vi "DAQ - 1-7 Modules - SubVI.vi"(11 "array":dbl[](array[numeric])) -> (3 "output array":dbl[](array[numeric]))   [LabVIEW 2015]
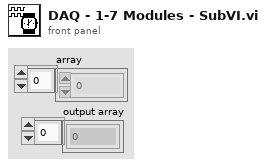
[diagram p1: front panel]
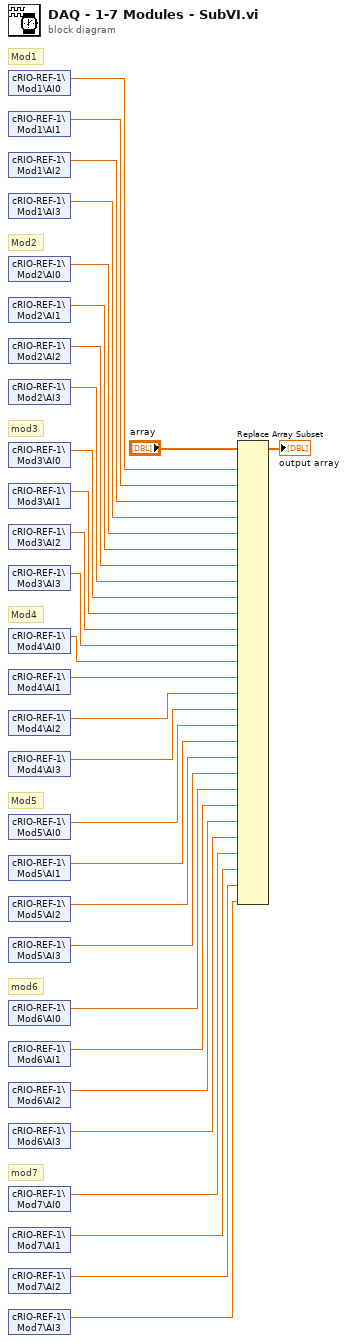
[diagram p0: block diagram]
diagram:
  # "mod3"
  # "Mod1"
  # "Mod2"
  # "mod6"
  # "mod7"
  # "Mod4"
  # "Mod5"
  n1 = shared-variable "cRIO-REF-1\\Mod1\\AI0"() -> (w1:dbl)  [unwired: 1 in, 1 out]
  n2 = shared-variable "cRIO-REF-1\\Mod1\\AI1"() -> (w2:dbl)  [unwired: 1 in, 1 out]
  n3 = shared-variable "cRIO-REF-1\\Mod1\\AI2"() -> (w3:dbl)  [unwired: 1 in, 1 out]
  n4 = shared-variable "cRIO-REF-1\\Mod1\\AI3"() -> (w4:dbl)  [unwired: 1 in, 1 out]
  n5 = shared-variable "cRIO-REF-1\\Mod2\\AI0"() -> (w5:dbl)  [unwired: 1 in, 1 out]
  n6 = shared-variable "cRIO-REF-1\\Mod2\\AI1"() -> (w6:dbl)  [unwired: 1 in, 1 out]
  n7 = shared-variable "cRIO-REF-1\\Mod2\\AI2"() -> (w7:dbl)  [unwired: 1 in, 1 out]
  n8 = shared-variable "cRIO-REF-1\\Mod2\\AI3"() -> (w8:dbl)  [unwired: 1 in, 1 out]
  n9 = shared-variable "cRIO-REF-1\\Mod3\\AI0"() -> (w9:dbl)  [unwired: 1 in, 1 out]
  n10 = shared-variable "cRIO-REF-1\\Mod3\\AI1"() -> (w10:dbl)  [unwired: 1 in, 1 out]
  n11 = shared-variable "cRIO-REF-1\\Mod3\\AI2"() -> (w11:dbl)  [unwired: 1 in, 1 out]
  n12 = shared-variable "cRIO-REF-1\\Mod3\\AI3"() -> (w12:dbl)  [unwired: 1 in, 1 out]
  n13 = shared-variable "cRIO-REF-1\\Mod4\\AI0"() -> (w26:dbl)  [unwired: 1 in, 1 out]
  n14 = shared-variable "cRIO-REF-1\\Mod4\\AI1"() -> (w25:dbl)  [unwired: 1 in, 1 out]
  n15 = shared-variable "cRIO-REF-1\\Mod4\\AI2"() -> (w24:dbl)  [unwired: 1 in, 1 out]
  n16 = shared-variable "cRIO-REF-1\\Mod4\\AI3"() -> (w23:dbl)  [unwired: 1 in, 1 out]
  n17 = shared-variable "cRIO-REF-1\\Mod5\\AI0"() -> (w30:dbl)  [unwired: 1 in, 1 out]
  n18 = shared-variable "cRIO-REF-1\\Mod5\\AI1"() -> (w29:dbl)  [unwired: 1 in, 1 out]
  n19 = shared-variable "cRIO-REF-1\\Mod5\\AI2"() -> (w28:dbl)  [unwired: 1 in, 1 out]
  n20 = shared-variable "cRIO-REF-1\\Mod5\\AI3"() -> (w27:dbl)  [unwired: 1 in, 1 out]
  n21 = shared-variable "cRIO-REF-1\\Mod6\\AI0"() -> (w20:dbl)  [unwired: 1 in, 1 out]
  n22 = shared-variable "cRIO-REF-1\\Mod6\\AI1"() -> (w19:dbl)  [unwired: 1 in, 1 out]
  n23 = shared-variable "cRIO-REF-1\\Mod6\\AI2"() -> (w18:dbl)  [unwired: 1 in, 1 out]
  n24 = shared-variable "cRIO-REF-1\\Mod6\\AI3"() -> (w17:dbl)  [unwired: 1 in, 1 out]
  n25 = shared-variable "cRIO-REF-1\\Mod7\\AI0"() -> (w16:dbl)  [unwired: 1 in, 1 out]
  n26 = shared-variable "cRIO-REF-1\\Mod7\\AI1"() -> (w15:dbl)  [unwired: 1 in, 1 out]
  n27 = shared-variable "cRIO-REF-1\\Mod7\\AI2"() -> (w14:dbl)  [unwired: 1 in, 1 out]
  n28 = shared-variable "cRIO-REF-1\\Mod7\\AI3"() -> (w13:dbl)  [unwired: 1 in, 1 out]
  n29 = Replace Array Subset(array="array", new element #1=w1, new element #2=w2, new element #3=w3, new element #4=w4, new element #5=w5, new element #6=w6, new element #7=w7, new element #8=w8, new element #9=w9, new element #10=w10, new element #11=w11, new element #12=w12, new element #13=w26, new element #14=w25, new element #15=w24, new element #16=w23, new element #17=w30, new element #18=w29, new element #19=w28, new element #20=w27, new element #21=w20, new element #22=w19, new element #23=w18, new element #24=w17, new element #25=w16, new element #26=w15, new element #27=w14, new element #28=w13) -> (→"output array":dbl[])  [unwired: 28 in]
